vi "13.2 Particle Filter.vi"() -> ()   [LabVIEW 2016]
doc: "This example shows how to use the Edge Tool in NI Vision. The Edge Tool finds edges (or sharp transitions in the pixels values) along a given line or ROI profile. The Edge Tool is a precursor function to many of the gauging and inspection tasks. For example, the location of the edges found along a line profile across an object can interpreted as the boundaries of the object whose dimensions have to be measured for a gauging application or the presence of a crack in the surface of an object for an inspection application."
uses:
  <vilib>/vision/NI_Vision_Development_Module.lvlib
panel:
  out "Particle Reports (Pixels)":T1(array[cluster]) {"Orientation" format="%.2f"; "Dimensions"."Height" format="%.2f"; "Dimensions"."Width" format="%.2f"; "Center of Mass"."Y" format="%.2f"; "Center of Mass"."X" format="%.2f"; "Bounding Rect"."Bottom" format="%.2f"; "Bounding Rect"."Right" format="%.2f"; "Bounding Rect"."Top" format="%.2f"; "Bounding Rect"."Left" format="%.2f"; "Number of Holes" format="%.2f"; "Area" format="%.2f"}
  in  "Selection Values":T3(array[cluster])=[{"Measurement Parameter"=35, "Range Lower Value"=2590.0, "Range Upper Value"=2641.0, "Range"=FALSE, "Measurement Type"=FALSE}, {"Measurement Parameter"=16, "Range Lower Value"=62.0, "Range Upper Value"=63.0, "Range"=FALSE, "Measurement Type"=FALSE}] {"Measurement Parameter" items=["Center of Mass X", "Center of Mass Y", "First Pixel X", "First Pixel Y", "Bounding Rect Left", "Bounding Rect Top", "Bounding Rect Right", "Bounding Rect Bottom", "Max Feret Diameter Start X", "Max Feret Diameter Start Y", "Max Feret Diameter End X", "Max Feret Diameter End Y", "Max Horiz. Segment Length Left", "Max Horiz. Segment Length Right", "Max Horiz. Segment Length Row", "-", "Bounding Rect Width", "Bounding Rect Height", "Bounding Rect Diagonal", "Perimeter", "Convex Hull Perimeter", "Holes' Perimeter", "Max Feret Diameter", "Equivalent Ellipse Major Axis", "Equivalent Ellipse Minor Axis", "Equivalent Ellipse Minor Axis (Feret)", "Equivalent Rect Long Side", "Equivalent Rect Short Side", "Equivalent Rect Diagonal", "Equivalent Rect Short Side (Feret)", "Average Horiz. Segment Length", "Average Vert. Segment Length", "Hydraulic Radius", "Waddel Disk Diameter", "-", "Area", "Holes' Area", "Particle & Holes' Area", "Convex Hull Area", "Image Area", "-", "Number of Holes", "Number of Horiz. Segments", "Number of Vert. Segments", "-", "Orientation", "Max Feret Diameter Orientation", "-", "% Area/Image Area", "% Area/(Particle & Holes' Area)", "Ratio of Equivalent Ellipse Axes", "Ratio of Equivalent Rect Sides", "-", "Elongation Factor", "Compactness Factor", "Heywood Circularity Factor", "Type Factor", "-", "Sum X", "Sum Y", "Sum XX", "Sum XY", "Sum YY", "Sum XXX", "Sum XXY", "Sum XYY", "Sum YYY", "-", "Moment of Inertia XX", "Moment of Inertia XY", "Moment of Inertia YY", "Moment of Inertia XXX", "Moment of Inertia XXY", "Moment of Inertia XYY", "Moment of Inertia YYY", "Norm. Moment of Inertia XX", "Norm. Moment of Inertia XY", "Norm. Moment of Inertia YY", "Norm. Moment of Inertia XXX", "Norm. Moment of Inertia XXY", "Norm. Moment of Inertia XYY", "Norm. Moment of Inertia YYY", "Hu Moment 1", "Hu Moment 2", "Hu Moment 3", "Hu Moment 4", "Hu Moment 5", "Hu Moment 6", "Hu Moment 7"]; "Range Lower Value" format="%.2f"; "Range Upper Value" format="%.2f"}
  in  "Tab":enum32{"Src ", "Bin", "Selected"}(tab)=enum."Selected"
  out "Src":T4(plugin-control)
  out "Bin":T4(plugin-control)
  out "Dst":T4(plugin-control)
  in  "Threshold":cluster{"Lower\nValue":sgl, "Upper\nValue":sgl}={"Lower\nValue"=0.0, "Upper\nValue"=210.0}
  in  "Stop":bool
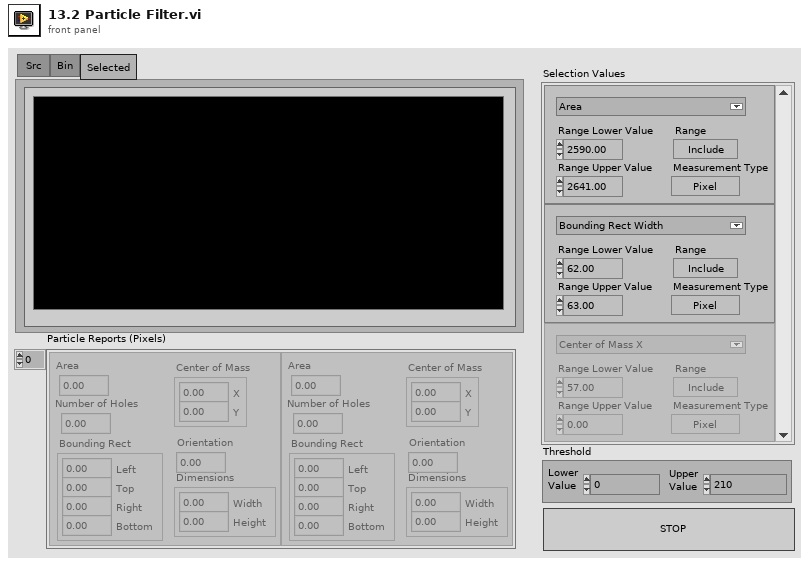
[diagram p1: front panel]
types:
  T1 = cluster{"Area":dbl, "Number of Holes":dbl, "Bounding Rect":cluster{"Left":dbl, "Top":dbl, "Right":dbl, "Bottom":dbl}, "Center of Mass":cluster{"X":dbl, "Y":dbl}, "Orientation":dbl, "Dimensions":cluster{"Width":dbl, "Height":dbl}}[]
  T2 = typedef "Particle Parameters" = i32
  T3 = cluster{"Measurement Parameter":T2, "Range Lower Value":dbl, "Range Upper Value":dbl, "Range":bool, "Measurement Type":bool}[]
  T4 = typedef "IMAQ Image.ctl" = refnum<image>
  T5 = cluster{"Threshold":cluster{"Lower\nValue":sgl, "Upper\nValue":sgl}, "Selection Values":cluster{"Measurement Parameter":T2, "Range Lower Value":dbl, "Range Upper Value":dbl, "Range":bool, "Measurement Type":bool}[]}
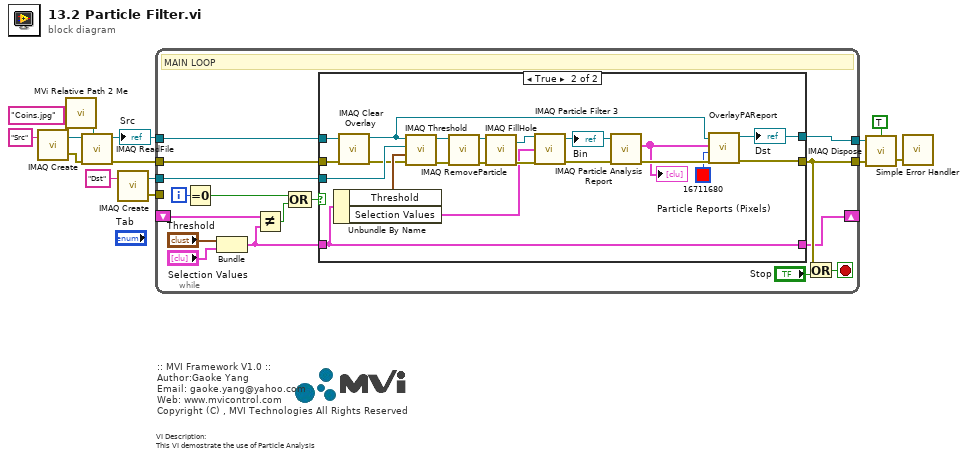
[diagram p0: block diagram]
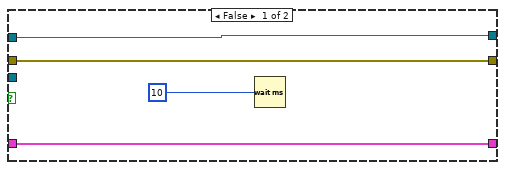
[diagram p2: hidden frame]
diagram:
  # "VI Description:\nThis VI demostrate the use of Particle Analysis"
  # ":: MVI Framework V1.0 ::\nAuthor:Gaoke Yang\nEmail: gaoke.yang@yahoo.com\nWeb: www.mvicontrol.com\nCopyright (C) , MVI Technologies All Rights Reserved"
  n1 = call "IMAQ Create"("Image Name"="Src") -> ("New Image"=w13:T4, "error out"=w12:errorcluster)  [unwired: 4 in]
  n2 = call "MVi Relative Path 2 Me.vi"("Relative Path"="Coins.jpg" ("name or relative path")) -> ("Appended Dir"=w8:path)  [unwired: 5 in, 1 out]
  n3 = call "IMAQ ReadFile"("File Path"=w8, "error in (no error)"=w12, "Image"=w13) -> ("error out"=w1:errorcluster, "Image Out"=w2:T4)  [unwired: 4 in, 3 out]
  "Src" <- w2
  n4 = call "IMAQ Create"("Image Name"="Dst") -> ("New Image"=w4:T4, "error out"=w3:errorcluster)  [unwired: 4 in]
  n5 = while "MAIN LOOP" {
    tunnel: w2 -> [w17]
    tunnel: w1 -> [w16]
    tunnel: [w27] -> w11
    tunnel: [w28] -> w10
    shift-right: [w24] -> _
    shift-left: _ -> [w22]
    tunnel: w4 -> [w18]
    tunnel: w3 -> [_]
    i -> [w26]
    stop <- w29 stop-if-true
    # "MAIN LOOP"
    n6 = Equal To 0?(x=w26) -> (x = 0?=w23:bool)
    n7 = Bundle("Threshold"="Threshold", "Selection Values"="Selection Values") -> (w20:T5)  [unwired: 1 in]
    n8 = Not Equal?(x=w22, y=w20) -> (x != y?=w21:bool)
    n9 = Compound Arithmetic op=OR(w23, w21) -> (w25:bool)
    n10 = case shown="True" w25 {
      tunnel: w16 -> [w33 w37]
      tunnel: w17 -> [w34 w38]
      tunnel: [w34 w39] -> w28
      tunnel: [w33 w43] -> w27
      tunnel: [w32 w55] -> w24
      tunnel: w20 -> [w32 w55]
      tunnel: w18 -> [_ w53]
      frame False {
        n11 = Wait (ms)(milliseconds to wait=u32 10) -> ()  [unwired: 1 out]
      }
      frame True {
        n12 = Unbundle By Name(w55) -> ("Threshold"=w54:cluster{"Lower\nValue":sgl, "Upper\nValue":sgl}, "Selection Values"=w46:T3)
        n13 = call "IMAQ Clear Overlay"("error in (no error)"=w37, "Image"=w38) -> ("error out"=w36:errorcluster, "Image Out"=w35:T4)  [unwired: 8 in]
        n14 = call "IMAQ Threshold"("error in (no error)"=w36, "Range"=w54, "Image Dst"=w53, "Image Src"=w35) -> ("error out"=w52:errorcluster, "Image Dst Out"=w51:T4)  [unwired: 2 in, 4 out]
        n15 = call "IMAQ RemoveParticle"("error in (no error)"=w52, "Image Src"=w51) -> ("error out"=w50:errorcluster, "Image Dst Out"=w49:T4)  [unwired: 8 in]
        n16 = call "IMAQ FillHole"("error in (no error)"=w50, "Image Src"=w49) -> ("error out"=w48:errorcluster, "Image Dst Out"=w47:T4)  [unwired: 4 in]
        n17 = call "IMAQ Particle Filter 3"("Image Src"=w47, "Selection Values"=w46, "error in (no error)"=w48) -> ("Image Dst Out"=w40:T4, "error out"=w45:errorcluster)  [unwired: 10 in, 1 out]
        "Bin" <- w40
        n18 = call "IMAQ Particle Analysis Report"("error in (no error)"=w45, "Image"=w40) -> ("error out"=w44:errorcluster, "Particle Reports (Pixels)"=w42:T1)  [unwired: 4 in, 4 out]
        "Particle Reports (Pixels)" <- w42
        n19 = call "OverlayPAReport.vi"("error in"=w44, "Color"=u32 16711680, "Particle Reports (Pixels)"=w42, "Image"=w35) -> ("error out"=w43:errorcluster, "Image Out"=w39:T4)  [unwired: 6 in]
        "Dst" <- w39
      }
    }
    n20 = Or(x=w27, y="Stop") -> (x .or. y?=w29:bool)
  }
  n21 = call "IMAQ Dispose"("All Images? (No)"=TRUE, "Image"=w10, "error in (no error)"=w11) -> ("error out"=w7:errorcluster)  [unwired: 3 in]
  n22 = call <vilib>:"Simple Error Handler.vi"("error in (no error)"=w7) -> ()  [unwired: 4 in, 5 out]
